vi "WorkorderHandler_SetBadNo.vi"(8 "error in (no error)":errorcluster, 10 "BadNo":string, 11 "reference":T1) -> (0 "error out":errorcluster, 3 "duplicate reference":T1)   [LabVIEW 2011]
uses:
  DataStructures/WorkorderHandler_ObjectReference.ctl
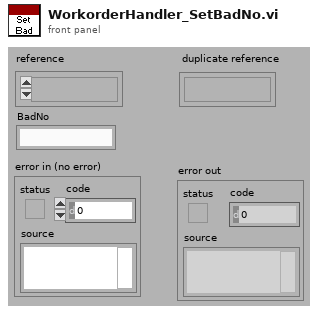
[diagram p1: front panel]
types:
  T1 = typedef "WorkorderHandler_ObjectReference.ctl" = refnum<k1>
  T2 = typedef "WorkorderHandler_ObjectData.ctl" = cluster{"Table":string[][], "Script":string, "Order":string, "No":string, "Time":dbl}
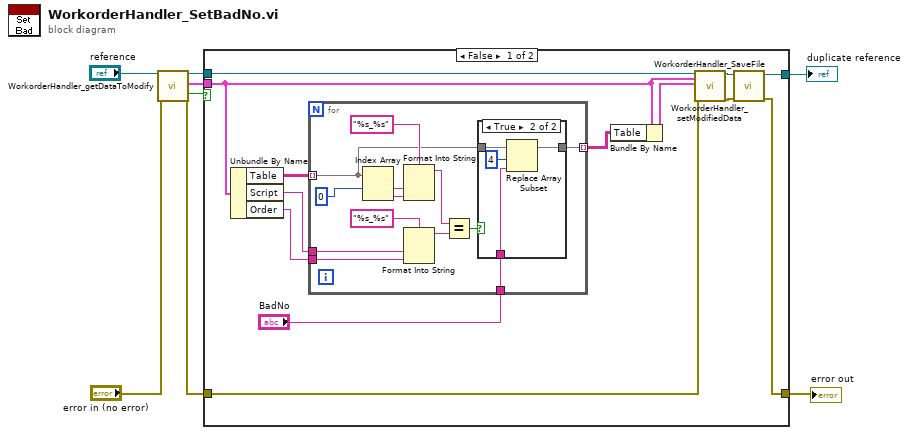
[diagram p0: block diagram]
diagram:
  n1 = call "WorkorderHandler_getDataToModify.vi"("reference"="reference", "error in (no error)"="error in (no error)") -> ("duplicate reference"=w4:T1, "data"=w7:T2, "timed out?"=w2:bool, "error out"=w3:errorcluster)  [unwired: 1 in, 13 out]
  n2 = case shown="False" w2 {
    tunnel: [w10 w41] -> w8
    tunnel: w7 -> [w15 _]
    tunnel: w4 -> [w21 w40]
    tunnel: w3 -> [w19 w41]
    tunnel: [w9 w40] -> w1
    frame False {
      n3 = Unbundle By Name(w15) -> ("Table"=w16:string[][], "Script"=w17:string, "Order"=w18:string)
      n4 = for {
        tunnel: w16 -> [w24] mode=indexing
        tunnel: w17 -> [w28]
        tunnel: w18 -> [w27]
        tunnel: [w23] -> w14 mode=indexing
        tunnel: "BadNo" -> [w22]
        n5 = Index Array(array=w24, index #1=0 ("index")) -> (element #1=w30:string, element #2=w29:string)  [unwired: 1 in]
        n6 = Format Into String(format string="%s_%s", w30, w29) -> (resulting string=w26:string)  [unwired: 2 in, 1 out]
        n7 = Format Into String(format string="%s_%s", w28, w27) -> (resulting string=w25:string)  [unwired: 2 in, 1 out]
        n8 = Equal?(x=w26, y=w25) -> (x = y?=w33:bool)
        n9 = case shown="True" w33 {
          tunnel: w24 -> [w35 w39]
          tunnel: [w35 w38] -> w23
          tunnel: w22 -> [_ w37]
          frame False {
          }
          frame True {
            n10 = Replace Array Subset(array=w39, new element=w37, index=4) -> (w38:string[])
          }
        }
      }
      n11 = Bundle By Name(cluster=w15, "Table"=w14) -> (w20:T2)
      n12 = call "WorkorderHandler_setModifiedData.vi"("reference"=w21, "data (unmodified)"=w15, "data"=w20, "error in (no error)"=w19) -> ("duplicate reference"=w12:T1, "error out"=w11:errorcluster)  [unwired: 14 out]
      n13 = call "WorkorderHandler_SaveFile.vi"("error in (no error)"=w11, "reference"=w12) -> ("error out"=w10:errorcluster, "duplicate reference"=w9:T1)  [unwired: 8 out]
    }
    frame True {
      # "Error or Timed Out"
    }
  }
  "error out" <- w8
  "duplicate reference" <- w1
